vi "eTdsBLE_InitDevice.vi"(2 "characteristicUUID":string="AA11", 3 "serviceUUID":string="AA10", 4 "NumEltDataArray":i32=6) -> (0 "error out":errorcluster, 1 "eTdsDevice Reference":refnum<k24>)   [LabVIEW 2013]
uses:
  D:/GitHub/GT-Bionics/TDS-HM/Labview Code/C# BLE Interface/eTDS BLE Interface/TdsBleInterface for LV/TdsForLV/TdsForLV/bin/TdsForLV.dll
  TdsForLV/TdsForLV/bin/TdsForLV.dll
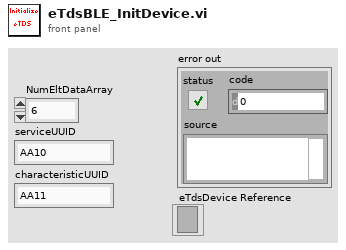
[diagram p1: front panel]
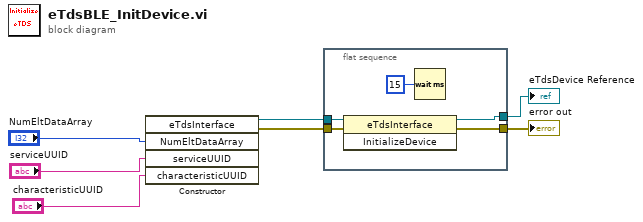
[diagram p0: block diagram]
diagram:
  n1 = constructor class="eTdsInterface"("NumEltDataArray"="NumEltDataArray", "serviceUUID"="serviceUUID", "characteristicUUID"="characteristicUUID") -> (reference out=w7:refnum<k24>, error out=w6:errorcluster)  [unwired: 3 in, 4 out]
  n2 = flat-sequence {
    tunnel: w7 -> [w12]
    tunnel: w6 -> [w11]
    tunnel: [w10] -> w5
    tunnel: [w9] -> w4
    frame #0 {
      n3 = invoke class="eTdsInterface" method="InitializeDevice"(reference=w12, error in=w11) -> (reference out=w10:refnum<k24>, error out=w9:errorcluster)  [unwired: 1 in, 1 out]
      n4 = Wait (ms)(milliseconds to wait=u32 15) -> ()  [unwired: 1 out]
    }
  }
  "error out" <- w4
  "eTdsDevice Reference" <- w5
